vi "Get position.vi"(8 "error in (no error)":errorcluster, 11 "Tomo in":refnum<class "Tomo.lvclass">) -> (0 "error out":errorcluster, 1 "Z position":dbl[unit], 2 "Y position":dbl[unit], 3 "Tomo out":refnum<class "Tomo.lvclass">, 4 "Angular position":dbl[unit], 5 "X position":dbl[unit])   [LabVIEW 2012, in "Tomo.lvclass"]
uses:
  Tomo.lvclass
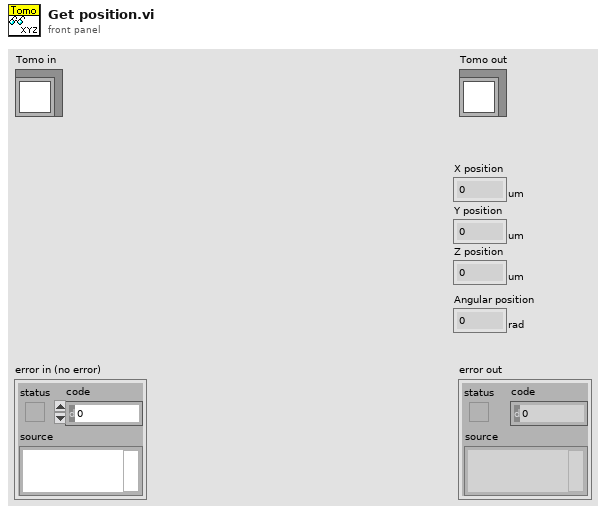
[diagram p1: front panel]
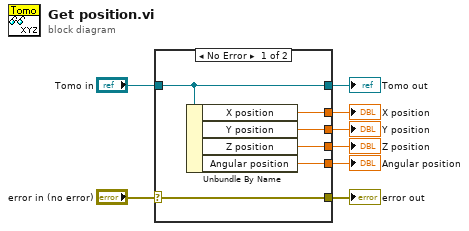
[diagram p0: block diagram]
diagram:
  n1 = case shown="No Error" "error in (no error)" {
    selector: "error in (no error)" -> [w14 w16]
    tunnel: [w14 w16] -> w7
    tunnel: [w13 w15] -> w5
    tunnel: "Tomo in" -> [w13 w15]
    tunnel: [w12 _] -> w4
    tunnel: [w11 _] -> w3
    tunnel: [w10 _] -> w2
    tunnel: [w9 _] -> w1
    frame No Error {
      n2 = Unbundle By Name(w13) -> ("X position"=w12:dbl[unit], "Y position"=w11:dbl[unit], "Z position"=w10:dbl[unit], "Angular position"=w9:dbl[unit])
    }
    frame Error {
    }
  }
  "error out" <- w7
  "Tomo out" <- w5
  "X position" <- w4
  "Y position" <- w3
  "Z position" <- w2
  "Angular position" <- w1
